vi "TDMS_strings to file 2.vi"(0 "Base path":path, 1 "Group Name":string="A", 2 "FileName":string, 3 "Interval":T1, 5 "Channel Names":string[](array[string]), 9 "Data":string[](array[string]), 11 "error in (no error)":errorcluster, 12 "Channel Units":string[](array[string]), 13 "property Metadata":variant[](array[variant])) -> (4 "file out":refnum<k34>, 15 "error out":errorcluster)   [LabVIEW 2019]
doc: "This SubVI manages the TDMS write process for data formatted into string arrays. On first run or after a specified interval, it will create a new TDMS file with a unique file name utilizing the date and time when the file is created. During the first run, it will populate the metadata and unit fields of the TDMS header. After a specified interval of data streaming to the file, it will be closed and the file extension will be changed from .tdms to .done. This is feature is to assure file transfer functions don't grab files that are being actively written to (LabVIEW's TDMS Open vi does not allow custom/alternate/temp file extensions). File write buffers are automatically flushed every 60 seconds to assure minimal data loss in the event of a power failure or program interruption. \n\n\nThis vi differs from version 1 by adding inputs for writing to the units column in the metadata page. Will replace version 1 once other code is updated.\n\n2020 NREL"
uses:
  Globals and Definitions/Enum_FileNewInterval.ctl
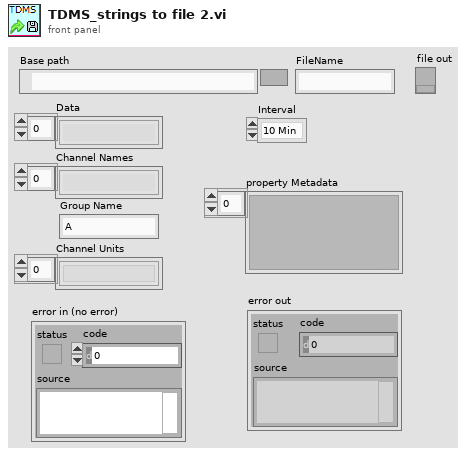
[diagram p1: front panel]
types:
  T1 = typedef "Enum_FileNewInterval.ctl" = enum16{"10 Min", "Hourly", "Daily", "Weekly", "Monthly"}
  T2 = enum16{"open", "open or create", "create or replace", "create", "open (read-only)"}
  T3 = typedef "LVDateTimeRec.ctl" = cluster{"fractional second":dbl, "second":i32, "minute":i32, "hour":i32, "day of month":i32, "month":i32, "year":i32, "day of week":i32, "day of year":i32, "DST":i32}
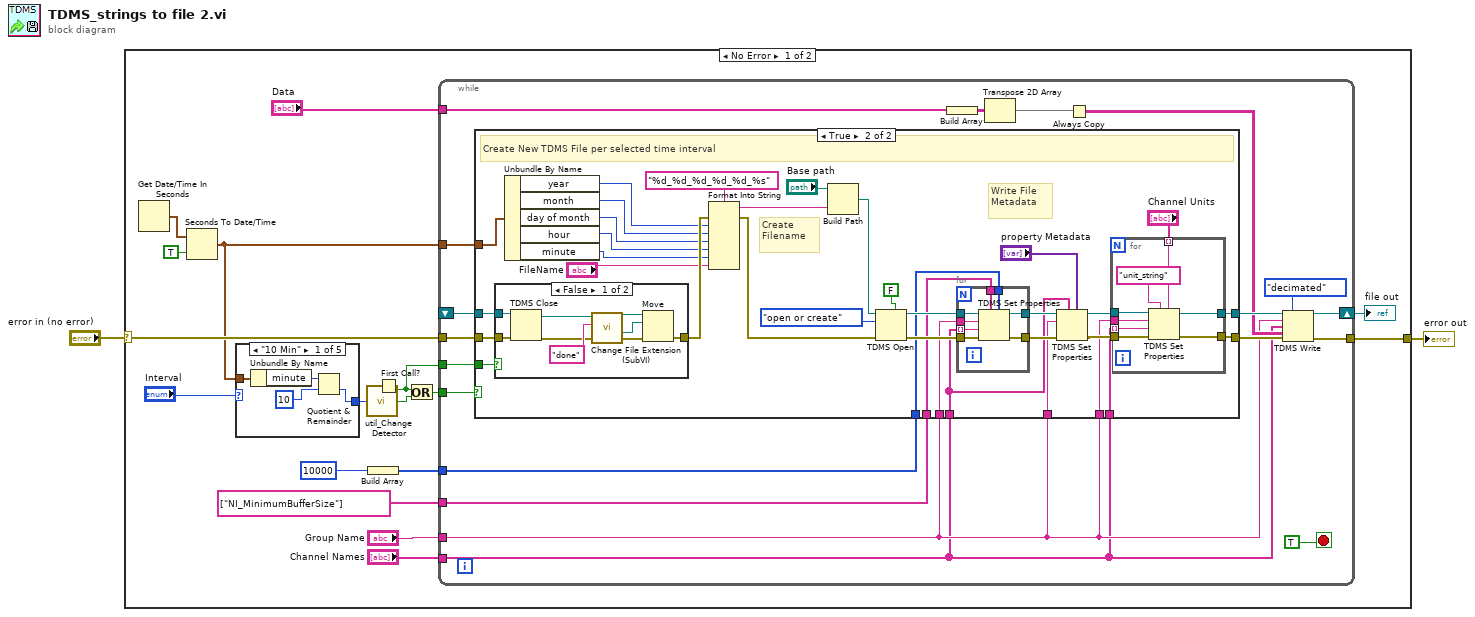
[diagram p0: block diagram]
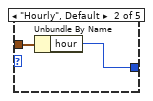
[diagram p2: hidden frame]
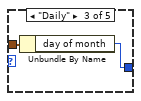
[diagram p3: hidden frame]
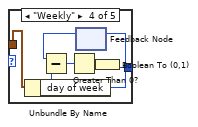
[diagram p4: hidden frame]
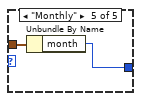
[diagram p5: hidden frame]
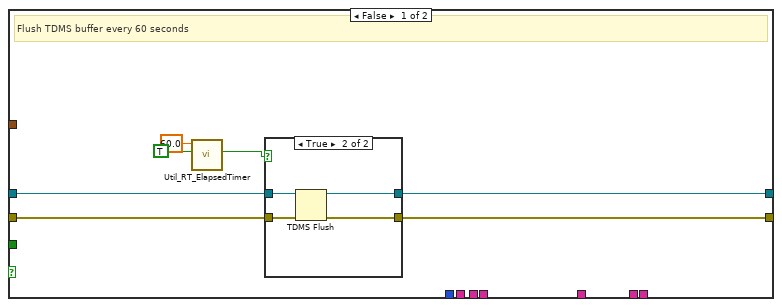
[diagram p6: hidden frame]
diagram:
  n1 = case shown="No Error" "error in (no error)" {
    selector: "error in (no error)" -> [w15 w128]
    tunnel: [w17 w128] -> w2
    frame No Error {
      n2 = Get Date/Time In Seconds() -> (seconds since 1Jan1904=w6:timestamp)
      n3 = Seconds To Date/Time(time stamp (now)=w6, to UTC (F)=TRUE) -> (date time rec=w5:T3)
      n4 = case shown="\"10 Min\"" "Interval" {
        tunnel: w5 -> [w23 w25 w27 w33 w35]
        tunnel: [w20 w24 w26 w28 w34] -> w3
        frame "10 Min" {
          n5 = Unbundle By Name(w23) -> ("minute"=w22:i32)
          n6 = Quotient & Remainder(x=w22, y=10) -> (floor(x/y)=w20:i32)  [unwired: 1 out]
        }
        frame "Hourly", Default {
          n7 = Unbundle By Name(w25) -> ("hour"=w24:i32)
        }
        frame "Daily" {
          n8 = Unbundle By Name(w27) -> ("day of month"=w26:i32)
        }
        frame "Weekly" {
          n9 = Unbundle By Name(w33) -> ("day of week"=w31:i32)
          n10 = feedback-in #1(w31) -> ()
          n11 = feedback #1() -> (w32:i32)  [unwired: 1 in]
          n12 = Subtract(x=w32, y=w31) -> (x-y=w30:i32)
          n13 = Greater Than 0?(x=w30) -> (x > 0?=w29:bool)
          n14 = Boolean To (0,1)(Boolean=w29) -> (0, 1=w28:i16)
        }
        frame "Monthly" {
          n15 = Unbundle By Name(w35) -> ("month"=w34:i32)
        }
      }
      n16 = call "util_Change Detector.vi"("value"=w3) -> ("changed?"=w4:bool)
      n17 = Build Array(10000) -> (w12:i32[])
      n18 = First Call?() -> (First Call?: T/F=w18:bool)
      n19 = Or(x=w18, y=w4) -> (x .or. y?=w19:bool)
      n20 = while {
        tunnel: w19 -> [w54]
        shift-right: [w52] -> w16
        shift-left: _ -> [w53]
        tunnel: w18 -> [w51]
        tunnel: "Data" -> [w45]
        tunnel: [w49] -> w17
        tunnel: w15 -> [w48]
        tunnel: w5 -> [w46]
        tunnel: w12 -> [w44]
        tunnel: string[] ["NI_MinimumBufferSize"] ("Channel Names") -> [w43]
        tunnel: "Group Name" -> [w37]
        tunnel: "Channel Names" -> [w36]
        stop <- TRUE stop-if-true
        n21 = case shown="True" w54 {
          tunnel: w53 -> [w61 w97]
          tunnel: w51 -> [_ w98]
          tunnel: [w58 w73] -> w42
          tunnel: w48 -> [w59 w96]
          tunnel: w46 -> [_ w93]
          tunnel: [w60 w74] -> w41
          tunnel: w44 -> [_ w90]
          tunnel: w43 -> [_ w89]
          tunnel: w37 -> [_ w76]
          tunnel: w36 -> [_ w80]
          tunnel: w37 -> [_ w78]
          tunnel: w37 -> [_ w71]
          tunnel: w36 -> [_ w70]
          frame False {
            # "Flush TDMS buffer every 60 seconds"
            n22 = call "Util_RT_ElapsedTimer.vi"("Auto Reset"=TRUE, "Target Time (s)"=60.0) -> ("Target\nReached"=w55:bool)  [unwired: 8 in, 1 out]
            n23 = case shown="True" w55 {
              tunnel: w61 -> [w63 w67]
              tunnel: [w63 w66] -> w60
              tunnel: w59 -> [w62 w65]
              tunnel: [w62 w64] -> w58
              frame False {
              }
              frame True {
                n24 = TDMS Flush(4:w65, 7:w67) -> (0:w64:errorcluster, 3:w66:refnum<k34>)
              }
            }
          }
          frame True {
            # "Create\nFilename"
            # "Write File\nMetadata"
            # "Create New TDMS File per selected time interval"
            n25 = case shown="False" w98 {
              tunnel: w97 -> [w126 _]
              tunnel: [w122 w127] -> w102
              tunnel: w96 -> [w125 w127]
              frame False {
                n26 = TDMS Close(8:w125, 11:w126) -> (0:w121:errorcluster, 3:w120:path)
                n27 = call "Change File Extension (SubVI).vi"("New Extension"="done", "appended path"=w120) -> ("New file path"=w124:path, "Original Path"=w119:path)  [unwired: 7 in, 1 out]
                n28 = Move(source path=w119, error in=w121, 10:w124) -> (error out=w122:errorcluster)  [unwired: 2 in, 2 out]
              }
              frame True {
              }
            }
            n29 = Unbundle By Name(w93) -> ("year"=w87:i32, "month"=w86:i32, "day of month"=w85:i32, "hour"=w84:i32, "minute"=w83:i32)
            n30 = Format Into String(format string="%d_%d_%d_%d_%d_%s", error in=w102, w87, w86, w85, w84, w83, "FileName") -> (resulting string=w88:string, error out=w94:errorcluster)  [unwired: 1 in]
            n31 = Build Path(base path="Base path", name or relative path=w88) -> (appended path=w100:path)
            n32 = TDMS Open(5:FALSE ("create index file? (T)"), 8:w94, 10:T2."open or create" ("operation (0:open)"), 11:w100) -> (0:w92:errorcluster, 3:w91:refnum<k34>)  [unwired: 3 in]
            n33 = for {
              tunnel: w91 -> [w118]
              tunnel: [w117] -> w82
              tunnel: w92 -> [w116]
              tunnel: [w115] -> w81
              tunnel: w89 -> [w114]
              tunnel: w90 -> [w113]
              tunnel: w76 -> [w112]
              tunnel: w80 -> [w111] mode=indexing
              n34 = TDMS Set Properties(5:w113, 7:w114, 8:w116, 9:w111, 10:w112, 11:w118) -> (0:w115:errorcluster, 3:w117:refnum<k34>)  [unwired: 2 out]
            }
            n35 = TDMS Set Properties(5:"property Metadata", 7:w80, 8:w81, 10:w78, 11:w82) -> (0:w72:errorcluster, 3:w75:refnum<k34>)  [unwired: 1 in, 2 out]
            n36 = for {
              tunnel: w71 -> [w108]
              tunnel: w75 -> [w110]
              tunnel: [w109] -> w74
              tunnel: [w107] -> w73
              tunnel: w72 -> [w106]
              tunnel: w70 -> [w105] mode=indexing
              tunnel: "Channel Units" -> [w103] mode=indexing
              n37 = TDMS Set Properties(5:w103, 7:"unit_string", 8:w106, 9:w105, 10:w108, 11:w110) -> (0:w107:errorcluster, 3:w109:refnum<k34>)  [unwired: 2 out]
            }
          }
        }
        n38 = Build Array(w45) -> (w40:string[][])
        n39 = Transpose 2D Array(2D array=w40) -> (transposed array=w39:string[][])
        n40 = Always Copy(1:w39) -> (0:w38:string[][])
        n41 = TDMS Write(0:w41, 1:enum16{"decimated", "interleaved"}."decimated" ("data layout (0:decimated)"), 5:w37, 7:w36, 9:w38, 11:w42) -> (4:w52:refnum<k34>, 15:w49:errorcluster)  [unwired: 2 out]
      }
      "file out" <- w16
    }
    frame Error {
    }
  }
  "error out" <- w2
